vi "Close comms.vi"(8 "error in (no error)":errorcluster, 11 "Program data":T1 {"Acq data"."Datos Osciloscopio"."Número Promedio" min=2 max=20; "Acq data"."Datos a Guardar In"."Posición Actual" format="%#_10f"; "Acq data"."Datos a Guardar In"."Posición Cero" format="%#_10f"; "Acq data"."Datos Bipolar/Unipolar"."Numero de lecturas" max=910098 step=1}) -> (0 "error out":errorcluster)   [LabVIEW 2020]
uses:
  <instrlib>/ZaberTSeries/ZaberTSeries.lvlib
  <instrlib>/Tektronix TDS 200 1000 2000 Series/Tektronix TDS 200 1000 2000 Series.lvlib
  Type Definitions/Datos Zaber.ctl
  Type Definitions/parametros motores.ctl
  Type Definitions/Datos a Guardar.ctl
  Type Definitions/datos osciloscopio.ctl
  H:/Mi unidad/Departamento de Ingenieria/Investigadores/Gabriel Ramos/Proyecto Monturas v13/LV Source/Type Definitions/Tipos de montura.ctl
  Type Definitions/Asistente de adquisicion Cluster.ctl
  Type Definitions/Program data.ctl
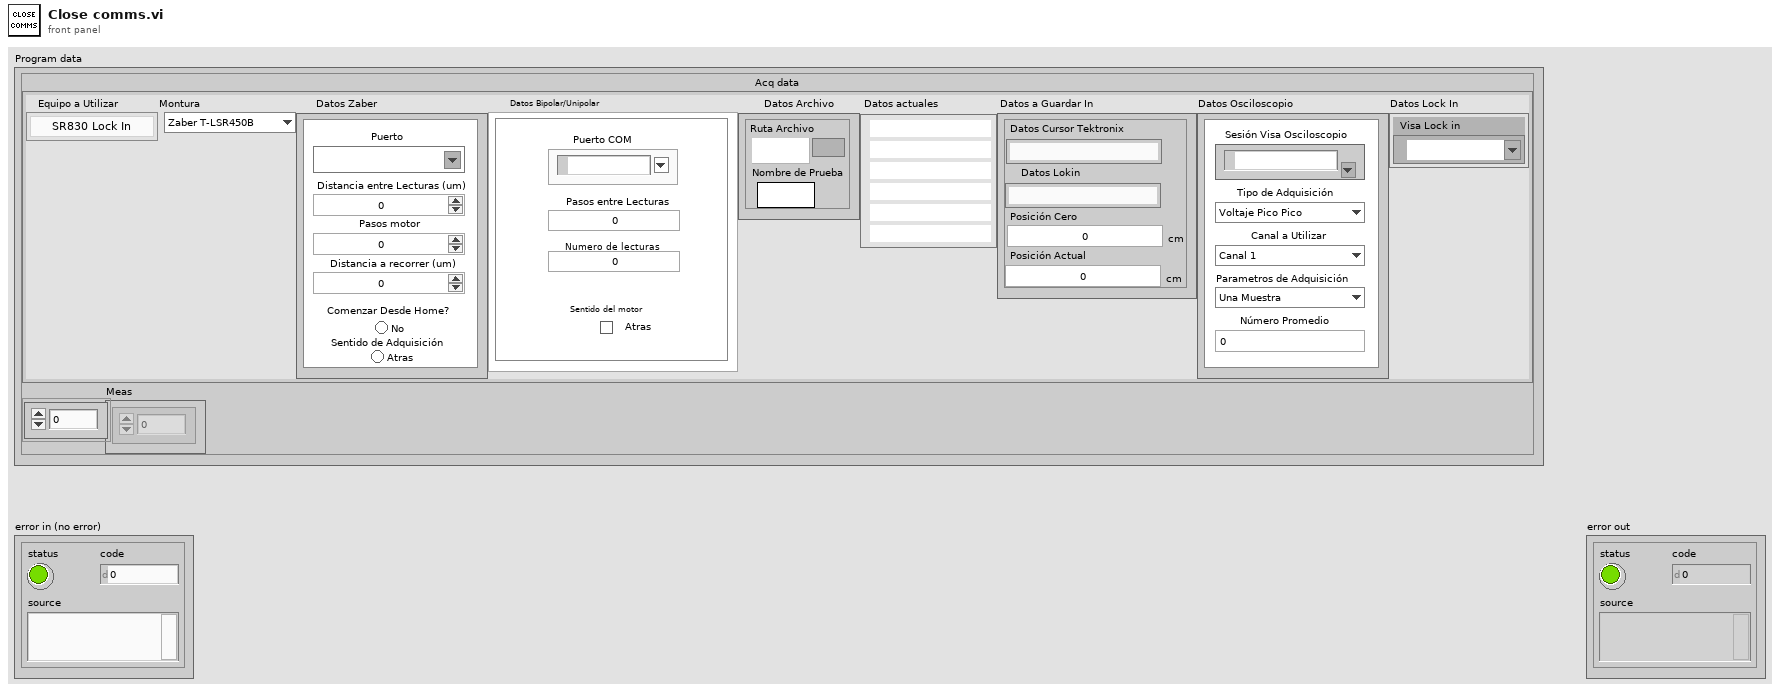
[diagram p1: front panel]
types:
  T1 = typedef "Program data.ctl" = cluster{"Acq data":T2, "Meas":dbl[]}
  T2 = typedef "Asistente de adquisicion Cluster.ctl" = cluster{"Equipo a Utilizar":enum16{"SR830 Lock In", "TDS 2012B Osciloscope"}, "Montura":T3, "Datos Zaber":T4, "Datos Bipolar/Unipolar":T5, "Datos Archivo":cluster{"Ruta Archivo":path, "Nombre de Prueba":string}, "Datos actuales":cluster{"Montura":string, "Equipo":string, "Posición Actual":string, "Distancia Total a recorrer":string, "distancia Entre lecturas":string, "Pasos entre lecturas":string}, "Datos a Guardar In":T6, "Datos Osciloscopio":T7, "Datos Lock In":cluster{"Visa Lock in":refnum<visa-resource-name>}}
  T3 = typedef "Tipos de montura.ctl" = enum16{"Zaber T-LSR450B", "Zaber-T-LSR300B", "Zaber-T-LSRxxx", "Motor Bipolar", "Motor Unipolar"}
  T4 = typedef "Datos Zaber.ctl" = cluster{"Sentido de Adquisición":bool, "Comenzar Desde Home?":bool, "Distancia a recorrer (um)":dbl, "Pasos motor":i32, "Distancia entre Lecturas (um)":dbl, "Puerto":refnum<visa-resource-name>}
  T5 = typedef "parametros motores.ctl" = cluster{"Puerto COM":refnum<visa-resource-name>, "Pasos entre Lecturas":u16, "Numero de lecturas":u32, "Sentido del motor":bool}
  T6 = typedef "Datos a Guardar.ctl" = cluster{"Datos Cursor Tektronix":string, "Datos Lokin":string, "Posición Cero":dbl[unit], "Posición Actual":dbl[unit]}
  T7 = typedef "datos osciloscopio.ctl" = cluster{"Sesión Visa Osciloscopio":refnum<visa-resource-name>, "Tipo de Adquisición":enum16{"Voltaje Pico Pico", "Voltaje RMS", "Cursor Tiempo"}, "Canal a Utilizar":enum16{"Canal 1", "Canal 2", "Canal 1 y 2"}, "Parametros de Adquisición":enum16{"Una Muestra", "Promedio"}, "Número Promedio":i32}
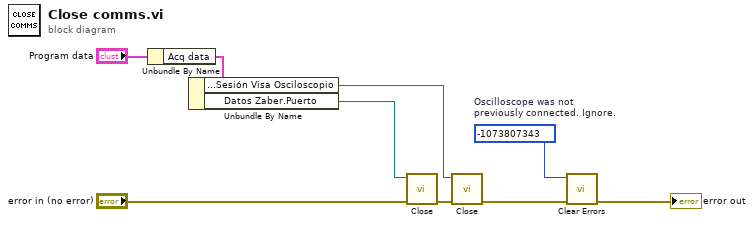
[diagram p0: block diagram]
diagram:
  w1 = -1073807343  # Oscilloscope was not  previously connected. Ignore.
  n1 = Unbundle By Name("Program data") -> ("Acq data"=w7:T2)
  n2 = Unbundle By Name(w7) -> ("Datos Osciloscopio.Sesión Visa Osciloscopio"=w9:refnum<visa-resource-name>, "Datos Zaber.Puerto"=w8:refnum<visa-resource-name>)
  n3 = call <instrlib>:"Close.vi"("error in (no error)"="error in (no error)", "VISA resource name"=w8) -> ("error out"=w4:errorcluster)  [unwired: 8 in, 1 out]
  n4 = call <instrlib>:"Close.vi"("error in (no error)"=w4, "VISA resource name"=w9) -> ("error out"=w5:errorcluster)  [unwired: 9 in]
  n5 = call <vilib>:"Clear Errors.vi"("error in (no error)"=w5, "specific error code to clear (0: all)"=w1) -> ("error out"=→"error out":errorcluster)  [unwired: 4 in, 1 out]
